vi "APP_Byte2Bit.vi"(11 "input byte stream":u8[](array[numeric])) -> (3 "output bit stream":i8[](array[numeric]))   [LabVIEW 2018]
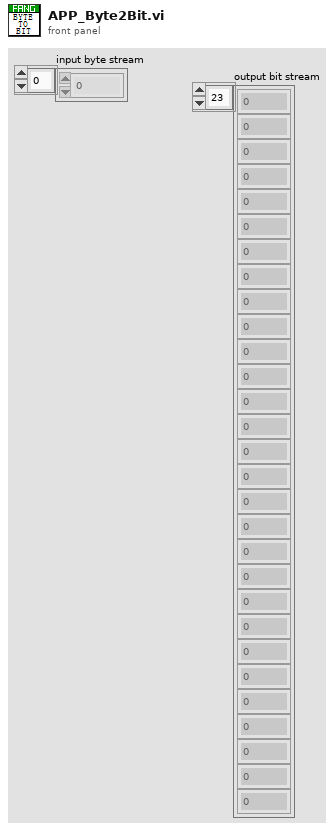
[diagram p1: front panel]
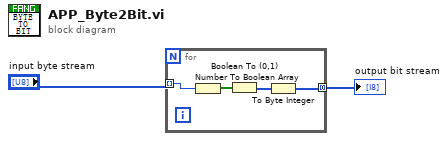
[diagram p0: block diagram]
diagram:
  n1 = for {
    tunnel: "input byte stream" -> [w6] mode=indexing
    tunnel: [w3] -> w1 mode=concatenating
    n2 = Number To Boolean Array(number=w6) -> (Boolean array=w5:bool[])
    n3 = Boolean To (0,1)(Boolean=w5) -> (0, 1=w4:i16[])
    n4 = To Byte Integer(number=w4) -> (8bit integer=w3:i8[])
  }
  "output bit stream" <- w1
